vi "FlatToRichni_measurementlink_pinmap_v1_QueryResourceAccessInformationResponse.vi"(5 "OutputClusterType":T1, 11 "InputCluster":T6) -> (3 "OutputCluster":T1)   [LabVIEW 2020, in "MeasurementLink Pin Map Client.lvlib"]
uses:
  MeasurementLink Pin Map Client.lvlib
  ni_measurementlink_pinmap_v1_QueryResourceAccessInformationResponse_Flat.ctl
  ni_measurementlink_pinmap_v1_ResourceAccessInformation_Flat.ctl
  ni_measurementlink_pinmap_v1_ChannelMapping_Flat.ctl
  ni_measurementlink_pinmap_v1_QueryResourceAccessInformationResponse_GroupMappingsEntry_Flat.ctl
  ni_measurementlink_pinmap_v1_ResolvedPinsOrRelays_Flat.ctl
  ni_measurementlink_pinmap_v1_QueryResourceAccessInformationResponse.ctl
  ni_measurementlink_pinmap_v1_ResourceAccessInformation.ctl
  ni_measurementlink_pinmap_v1_ChannelMapping.ctl
  ni_measurementlink_pinmap_v1_QueryResourceAccessInformationResponse_GroupMappingsEntry.ctl
  ni_measurementlink_pinmap_v1_ResolvedPinsOrRelays.ctl
  FlatToRichni_measurementlink_pinmap_v1_ChannelMapping.vi
  FlatToRichni_measurementlink_pinmap_v1_ResolvedPinsOrRelays.vi
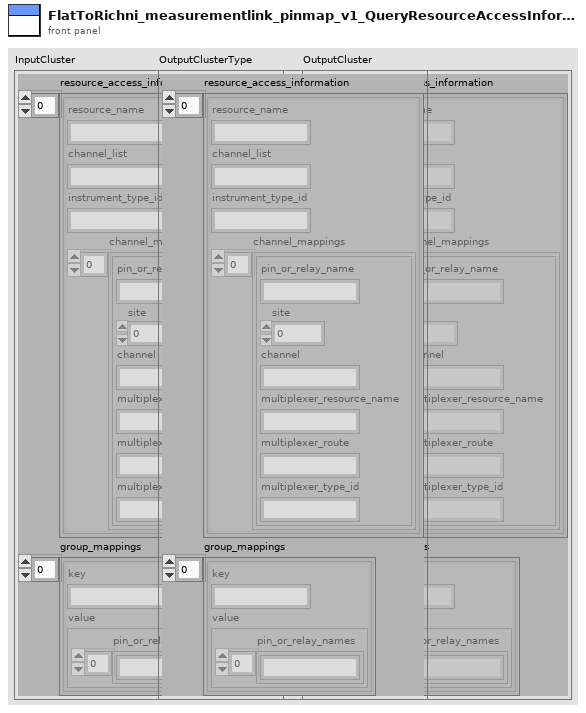
[diagram p1: front panel]
types:
  T1 = typedef "MeasurementLink Pin Map Client.lvlib/ni_measurementlink_pinmap_v1_QueryResourceAccessInformationResponse.ctl" = cluster{"resource_access_information":T2[], "group_mappings":T4[]}
  T2 = typedef "MeasurementLink Pin Map Client.lvlib/ni_measurementlink_pinmap_v1_ResourceAccessInformation.ctl" = cluster{"resource_name":string, "channel_list":string, "instrument_type_id":string, "channel_mappings":T3[]}
  T3 = typedef "MeasurementLink Pin Map Client.lvlib/ni_measurementlink_pinmap_v1_ChannelMapping.ctl" = cluster{"pin_or_relay_name":string, "site":i32, "channel":string, "multiplexer_resource_name":string, "multiplexer_route":string, "multiplexer_type_id":string}
  T4 = typedef "MeasurementLink Pin Map Client.lvlib/ni_measurementlink_pinmap_v1_QueryResourceAccessInformationResponse_GroupMappingsEntry.ctl" = cluster{"key":string, "value":T5}
  T5 = typedef "MeasurementLink Pin Map Client.lvlib/ni_measurementlink_pinmap_v1_ResolvedPinsOrRelays.ctl" = cluster{"pin_or_relay_names":string[]}
  T6 = typedef "MeasurementLink Pin Map Client.lvlib/ni_measurementlink_pinmap_v1_QueryResourceAccessInformationResponse_Flat.ctl" = cluster{"resource_access_information":T7[], "group_mappings":T9[]}
  T7 = typedef "MeasurementLink Pin Map Client.lvlib/ni_measurementlink_pinmap_v1_ResourceAccessInformation_Flat.ctl" = cluster{"resource_name":string, "channel_list":string, "instrument_type_id":string, "channel_mappings":T8[]}
  T8 = typedef "MeasurementLink Pin Map Client.lvlib/ni_measurementlink_pinmap_v1_ChannelMapping_Flat.ctl" = cluster{"pin_or_relay_name":string, "site":i32, "channel":string, "multiplexer_resource_name":string, "multiplexer_route":string, "multiplexer_type_id":string}
  T9 = typedef "MeasurementLink Pin Map Client.lvlib/ni_measurementlink_pinmap_v1_QueryResourceAccessInformationResponse_GroupMappingsEntry_Flat.ctl" = cluster{"key":string, "value":T10}
  T10 = typedef "MeasurementLink Pin Map Client.lvlib/ni_measurementlink_pinmap_v1_ResolvedPinsOrRelays_Flat.ctl" = cluster{"pin_or_relay_names":string[]}
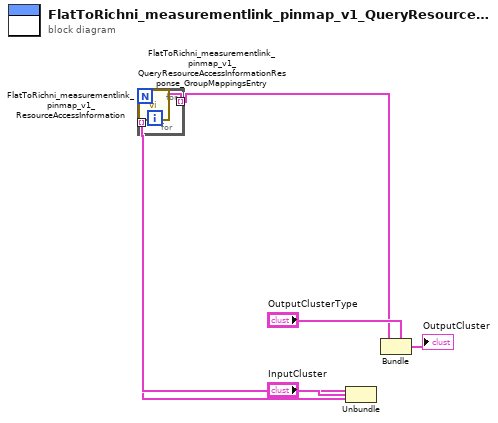
[diagram p0: block diagram]
diagram:
  n1 = Unbundle "Unbundle"("InputCluster") -> ("resource_access_information"=w4:T7[], "group_mappings"=w2:T9[])
  n2 = for {
    tunnel: w2 -> [w9] mode=indexing
    tunnel: [w8] -> w1 mode=indexing
    n3 = call "FlatToRichni_measurementlink_pinmap_v1_QueryResourceAccessInformationResponse_GroupMappingsEntry.vi"("InputCluster"=w9) -> ("OutputCluster"=w8:T4)  [unwired: 10 in]
  }
  n4 = for {
    tunnel: w4 -> [w11] mode=indexing
    tunnel: [w10] -> w3 mode=indexing
    n5 = call "FlatToRichni_measurementlink_pinmap_v1_ResourceAccessInformation.vi"("InputCluster"=w11) -> ("OutputCluster"=w10:T2)  [unwired: 10 in]
  }
  n6 = Bundle "Bundle"(cluster="OutputClusterType", "resource_access_information"=w3, "group_mappings"=w1) -> (→"OutputCluster":T1)
